vi "BT-Android_AE_sub.vi"(3 "port":u32=57600, 4 "file path (dialog if empty)":path=path "E:/测试数据/新芯片", 5 "mode":T1, 6 "timeout (10sec)":u32=10000, 7 "End Write on Termination Character?":bool, 8 "error in (no error)":errorcluster, 9 "存盘":bool, 10 "send data":string, 11 "VISA resource name":refnum<visa-resource-name>="COM13") -> (0 "error IO":errorcluster, 2 "timeout?":bool=TRUE)   [LabVIEW 2016, in "BT-Android_interface.lvlib"]
uses:
  BT-Android_interface.lvlib
  mode.ctl
  <vilib>/Utility/file.llb/Write Delimited Spreadsheet (I64).vi
  <vilib>/Instr/_visa.llb/VISA Configure Serial Port (Instr).vi
panel:
  in  "Termination Character":u8=10 format="%.0x"
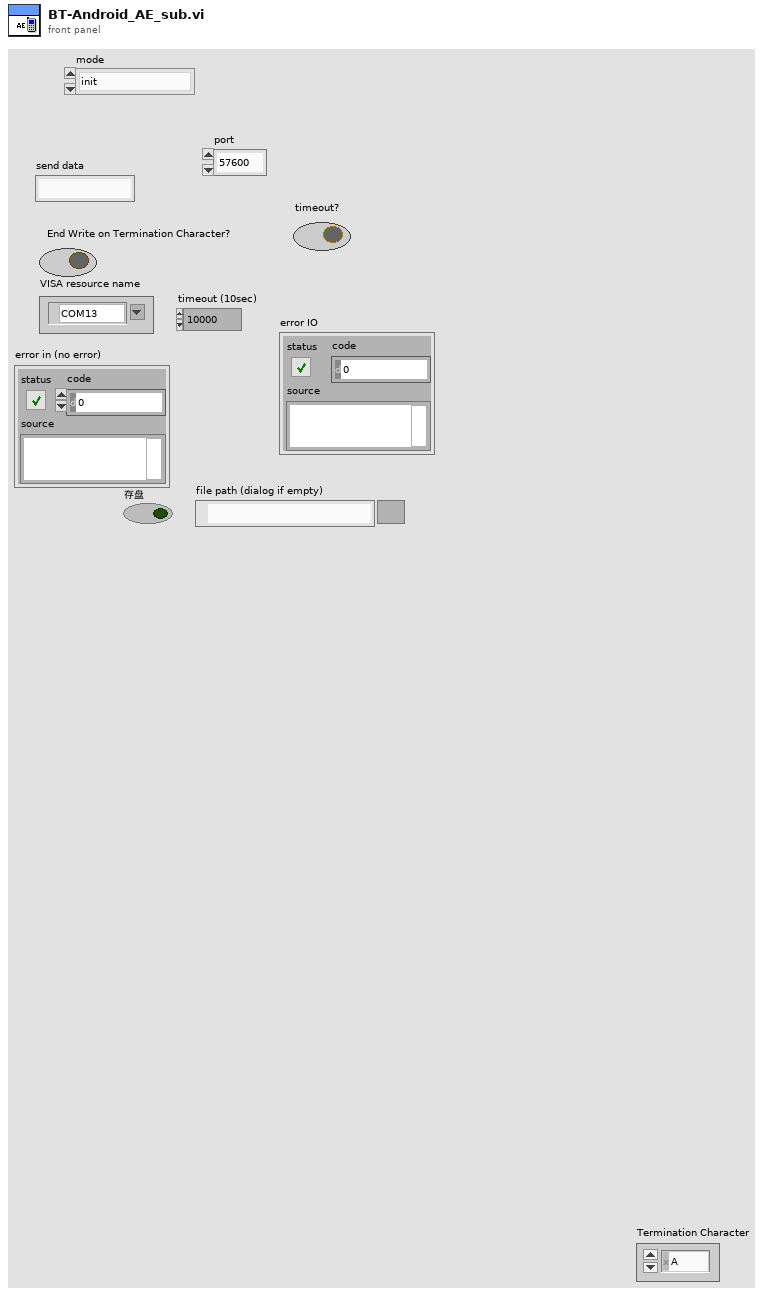
[diagram p1: front panel]
types:
  T1 = typedef "BT-Android_interface.lvlib/mode.ctl" = enum16{"init", "broadcast_data", "receive_data", "close"}
  T2 = enum16{"Standard", "Buffered", "CRLF", "Immediate"}
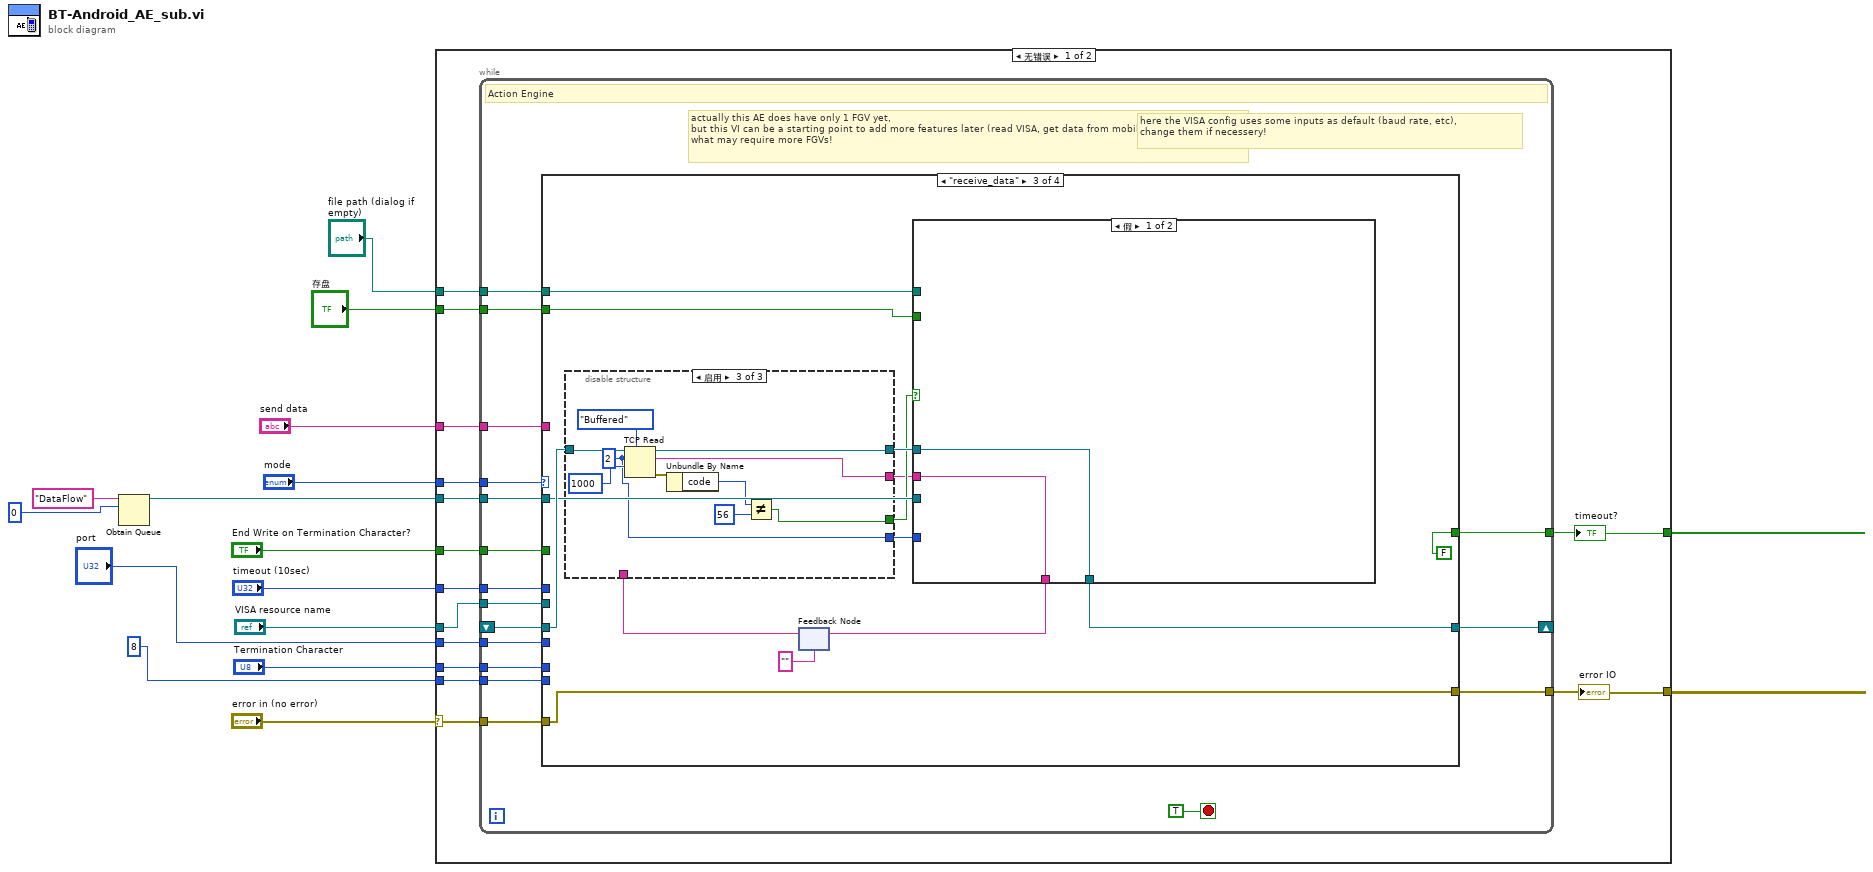
[diagram p0: block diagram]
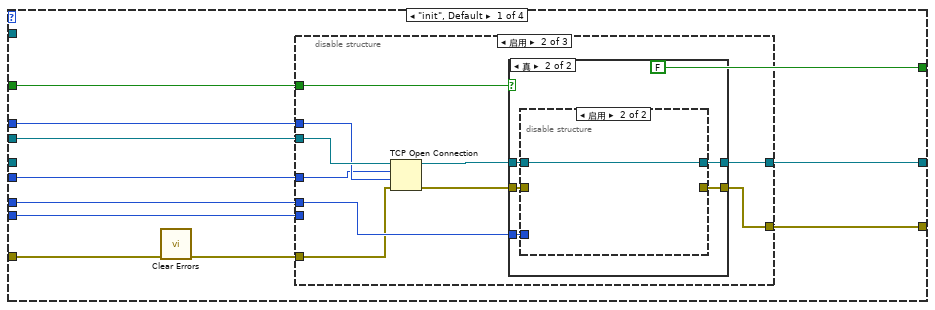
[diagram p2: hidden frame]
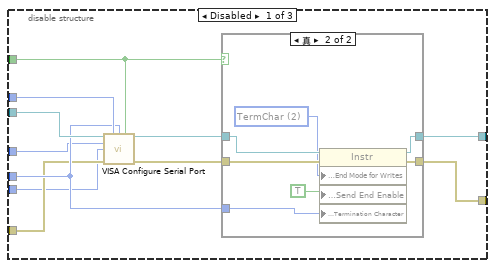
[diagram p3: hidden frame]
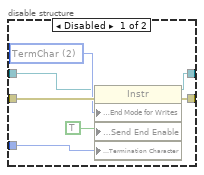
[diagram p6: hidden frame]
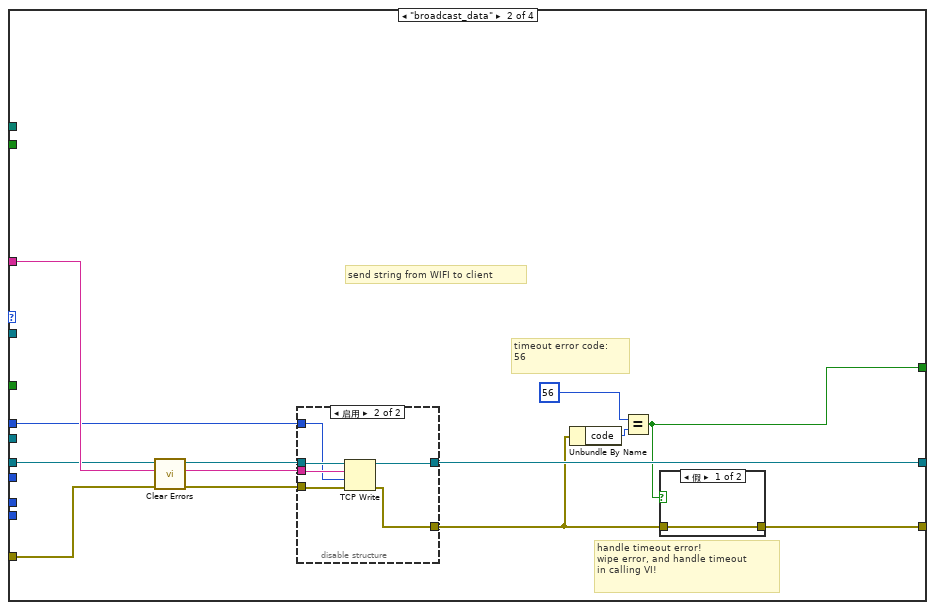
[diagram p8: hidden frame]
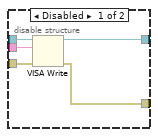
[diagram p9: hidden frame]
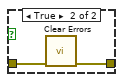
[diagram p10: hidden frame]
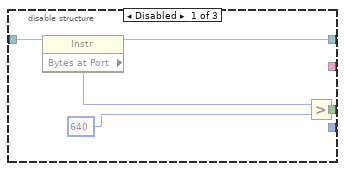
[diagram p11: hidden frame]
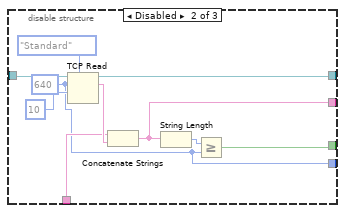
[diagram p12: hidden frame]
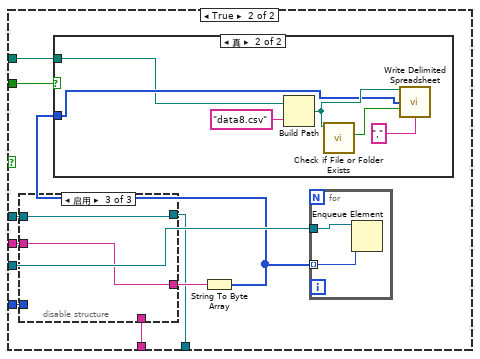
[diagram p13: hidden frame]
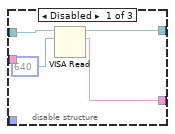
[diagram p14: hidden frame]
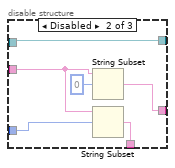
[diagram p15: hidden frame]
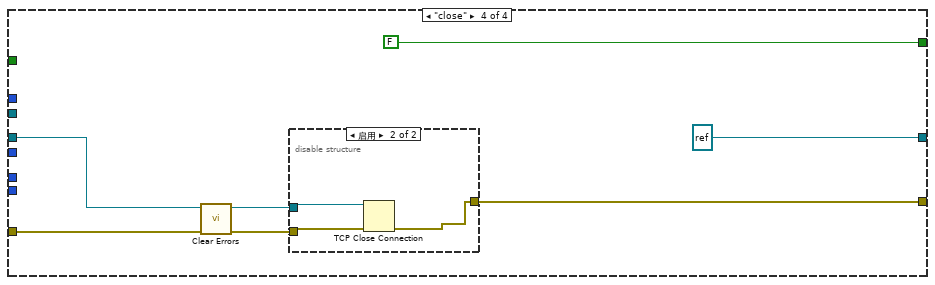
[diagram p17: hidden frame]
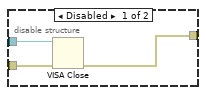
[diagram p18: hidden frame]
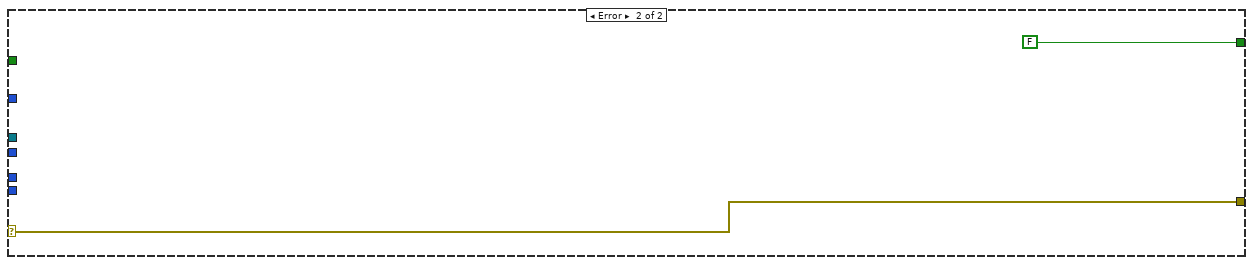
[diagram p19: hidden frame]
diagram:
  n1 = Obtain Queue(name (unnamed)="DataFlow", element data type=u8 0) -> (queue out=w5:refnum<queue>)  [unwired: 3 in, 2 out]
  n2 = case shown="无错误" "error in (no error)" {
    selector: "error in (no error)" -> [w30 w213]
    tunnel: [w26 w213] -> w15
    tunnel: "mode" -> [w29 _]
    tunnel: "End Write on Termination Character?" -> [w28 _]
    tunnel: "timeout (10sec)" -> [w27 _]
    tunnel: "VISA resource name" -> [w22 _]
    tunnel: "Termination Character" -> [w25 _]
    tunnel: "send data" -> [w24 _]
    tunnel: [w23 FALSE] -> w8
    tunnel: w5 -> [w21 _]
    tunnel: "port" -> [w20 _]
    tunnel: 8 -> [w19 _]
    tunnel: "存盘" -> [w18 _]
    tunnel: "file path (dialog if empty)" -> [w17 _]
    frame No Error {
      n3 = while {
        tunnel: w30 -> [w46]
        tunnel: w29 -> [w45]
        tunnel: w28 -> [w44]
        tunnel: w27 -> [w43]
        shift-right: [w42] -> _
        shift-left: _ -> [w36]
        tunnel: [w41] -> w26
        tunnel: w25 -> [w40]
        tunnel: w24 -> [w39]
        tunnel: [w38] -> w23
        tunnel: w22 -> [w37]
        tunnel: w21 -> [w35]
        tunnel: w20 -> [w34]
        tunnel: w19 -> [w33]
        tunnel: w18 -> [w32]
        tunnel: w17 -> [w31]
        stop <- TRUE stop-if-true
        # "here the VISA config uses some inputs as default (baud rate, etc),\nchange them if necessery!"
        # "actually this AE does have only 1 FGV yet, \nbut this VI can be a starting point to add more features later (read VISA, get data from mobile)\nwhat may require more FGVs!"
        # "Action Engine"
        n4 = case shown="\"receive_data\"" w45 {
          tunnel: w46 -> [w53 w114 w137 w205]
          tunnel: w44 -> [w51 _ _ _]
          tunnel: w43 -> [w58 w105 _ _]
          tunnel: w37 -> [w57 _ _ _]
          tunnel: [w56 w113 w138 refnum<k5> refnum ("connection ID")] -> w42
          tunnel: [w55 w111 w137 w204] -> w41
          tunnel: w40 -> [w54 _ _ _]
          tunnel: w39 -> [_ w112 _ _]
          tunnel: [FALSE w107 FALSE FALSE] -> w38
          tunnel: w36 -> [_ w106 w142 w201]
          tunnel: w35 -> [_ _ w140 _]
          tunnel: w34 -> [w50 _ _ _]
          tunnel: w33 -> [w49 _ _ _]
          tunnel: w32 -> [_ _ w136 _]
          tunnel: w31 -> [_ _ w135 _]
          frame "init", Default {
            n5 = call <vilib>:"Clear Errors.vi"("error in (no error)"=w53) -> ("error out"=w48:errorcluster)  [unwired: 5 in, 1 out]
            n6 = disable-structure shown="启用" {
              disable-tunnel: w58 -> [w67 w80 _]
              disable-tunnel: w57 -> [w66 w86 _]
              disable-tunnel: [w65 w85 _] -> w56
              disable-tunnel: [w64 w84 _] -> w55
              disable-tunnel: w54 -> [w63 w83 _]
              disable-tunnel: w48 -> [w62 w81 _]
              disable-tunnel: w51 -> [w61 w82 _]
              disable-tunnel: w50 -> [w60 w79 _]
              disable-tunnel: w49 -> [w59 _ _]
              frame Disabled {
                n7 = call-poly "VISA Configure Serial Port"("VISA resource name"=w66, "timeout (10sec)"=w67, "termination char\n(0xA = '\\n' = LF)"=w63, "Enable Termination\nChar (T)"=w61, "baud rate (9600)"=w60, "data bits (8)"=w59, "error in (no error)"=w62) -> ("VISA resource name out"=w68:refnum<visa-resource-name>, "error out"=w69:errorcluster)  [unwired: 3 in, 4 out]
                n8 = case shown="真" w61 {
                  tunnel: w68 -> [w70 w78]
                  tunnel: w69 -> [w71 w77]
                  tunnel: [w70 w76] -> w65
                  tunnel: [w71 w75] -> w64
                  tunnel: w63 -> [_ w73]
                  frame False {
                  }
                  frame True {
                    w74 = u16 2 items=["None", "LastBit", "TermChar", "Break"] ("Serial Settings:Serial End Mode for Writes")
                    n9 = property class="Instr"(reference=w78, error in=w77, "Serial Settings:End Mode for Writes"=w74, "Message Based Settings:Send End Enable"=TRUE, "Message Based Settings:Termination Character"=w73) -> (reference out=w76:refnum<visa-resource-name>, error out=w75:errorcluster)
                  }
                }
              }
              frame Enabled {
                n10 = TCP Open Connection(address=w86, remote port or service name=w79, timeout ms (60000)=w80, error in (no error)=w81) -> (connection ID=w87:refnum<k5>, error out=w88:errorcluster)  [unwired: 1 in]
                n11 = case shown="真" w82 {
                  tunnel: w87 -> [w89 w91]
                  tunnel: w88 -> [w90 w95]
                  tunnel: [w89 w94] -> w85
                  tunnel: [w90 w93] -> w84
                  tunnel: w83 -> [_ w92]
                  frame False {
                  }
                  frame True {
                    n12 = disable-structure shown="启用" {
                      disable-tunnel: w95 -> [w102 _]
                      disable-tunnel: [w101 w103] -> w94
                      disable-tunnel: [w100 _] -> w93
                      disable-tunnel: w92 -> [w98 _]
                      disable-tunnel: w91 -> [w96 w103]
                      frame Disabled {
                        w99 = u16 2 items=["None", "LastBit", "TermChar", "Break"] ("Serial Settings:Serial End Mode for Writes")
                        n13 = property class="Instr"(reference=w96, error in=w102, "Serial Settings:End Mode for Writes"=w99, "Message Based Settings:Send End Enable"=TRUE, "Message Based Settings:Termination Character"=w98) -> (reference out=w101:refnum<visa-resource-name>, error out=w100:errorcluster)
                      }
                      frame Enabled {
                      }
                    }
                  }
                }
              }
              frame Disabled {
              }
            }
          }
          frame "broadcast_data" {
            # "send string from WIFI to client"
            # "handle timeout error!\nwipe error, and handle timeout\nin calling VI!"
            # "timeout error code:\n56"
            n14 = call <vilib>:"Clear Errors.vi"("error in (no error)"=w114) -> ("error out"=w104:errorcluster)  [unwired: 5 in, 1 out]
            n15 = disable-structure shown="启用" {
              disable-tunnel: w104 -> [w119 w124]
              disable-tunnel: [w118 w122] -> w113
              disable-tunnel: w112 -> [w117 w123]
              disable-tunnel: [w116 w121] -> w110
              disable-tunnel: w106 -> [w115 w125]
              disable-tunnel: w105 -> [_ w120]
              frame Disabled {
                n16 = VISA Write(VISA resource name=w115, write buffer=w117, error in (no error)=w119) -> (VISA resource name out=w118:refnum<visa-resource-name>, error out=w116:errorcluster)  [unwired: 1 out]
              }
              frame Enabled {
                n17 = TCP Write(connection ID=w125, data in=w123, error in (no error)=w124, 9:w120) -> (connection ID out=w122:refnum<k5>, error out=w121:errorcluster)  [unwired: 1 out]
              }
            }
            n18 = Unbundle By Name(w110) -> ("code"=w109:i32)
            n19 = Equal?(x=56 ("code"), y=w109) -> (x = y?=w107:bool)
            n20 = case shown="假" w107 {
              tunnel: w110 -> [w126 w128]
              tunnel: [w126 w127] -> w111
              frame False {
              }
              frame True {
                n21 = call <vilib>:"Clear Errors.vi"("error in (no error)"=w128) -> ("error out"=w127:errorcluster)  [unwired: 5 in, 1 out]
              }
            }
          }
          frame "receive_data" {
            n22 = feedback #1("") -> (w132:string)
            n23 = disable-structure shown="启用" {
              disable-tunnel: w142 -> [w147 w157 w167]
              disable-tunnel: [w146 w155 w165] -> w141
              disable-tunnel: [w143 w150 w159] -> w134
              disable-tunnel: w132 -> [_ w151 _]
              disable-tunnel: [_ w149 w162] -> w131
              disable-tunnel: [_ w148 w163] -> w130
              frame Disabled {
                n24 = property class="Instr"(reference=w147) -> (reference out=w146:refnum<visa-resource-name>, "Bytes at Port"=w145:u32)  [unwired: 1 in, 1 out]
                n25 = Greater?(x=w145, y=640) -> (0:w143:bool)
              }
              frame Disabled {
                w148 = 640 ("读取的字节")
                n26 = TCP Read(connection ID=w157, bytes to read=w148, 7:T2."Standard" ("模式（标准）"), 9:10 ("超时毫秒(25000)")) -> (connection ID out=w155:refnum<k5>, data out=w152:string)  [unwired: 1 in, 1 out]
                n27 = Concatenate Strings(w151, w152) -> (w149:string)
                n28 = String Length(string=w149) -> (length=w153:i32)
                n29 = Greater Or Equal?(x=w153, y=w148) -> (x >= y?=w150:bool)
              }
              frame Enabled {
                w163 = 2 ("读取的字节")
                n30 = TCP Read(connection ID=w167, bytes to read=w163, 7:T2."Buffered" ("模式（标准）"), 9:1000 ("超时毫秒(25000)")) -> (connection ID out=w165:refnum<k5>, data out=w162:string, error out=w161:errorcluster)  [unwired: 1 in]
                n31 = Unbundle By Name(w161) -> ("code"=w160:i32)
                n32 = Not Equal?(x=w160, y=56) -> (x != y?=w159:bool)
              }
            }
            n33 = case shown="假" w134 {
              tunnel: w141 -> [w169 w179]
              tunnel: w140 -> [_ w177]
              tunnel: [w169 w176] -> w138
              tunnel: w136 -> [_ w175]
              tunnel: w135 -> [_ w174]
              tunnel: w131 -> [w168 w172]
              tunnel: w130 -> [_ w171]
              tunnel: [w168 w170] -> w129
              frame False {
              }
              frame True {
                n34 = disable-structure shown="启用" {
                  disable-tunnel: w179 -> [w183 w189 w191]
                  disable-tunnel: [w182 w185 w190] -> w178
                  disable-tunnel: [w181 w189 w191] -> w176
                  disable-tunnel: w172 -> [_ w187 w190]
                  disable-tunnel: w171 -> [_ w186 _]
                  disable-tunnel: [_ w184 _] -> w170
                  frame Disabled {
                    n35 = VISA Read(VISA resource name=w183, byte count=640) -> (VISA resource name out=w181:refnum<visa-resource-name>, read buffer=w182:string)  [unwired: 1 in, 2 out]
                  }
                  frame Disabled {
                    n36 = String Subset(string=w187, offset (0)=0 ("偏移量(0)")) -> (substring=w185:string)  [unwired: 1 in]
                    n37 = String Subset(string=w187, offset (0)=w186) -> (substring=w184:string)  [unwired: 1 in]
                  }
                  frame Enabled {
                  }
                }
                n38 = String To Byte Array(string=w178) -> (unsigned byte array=w173:u8[])
                n39 = case shown="真" w175 {
                  tunnel: w173 -> [_ w193]
                  tunnel: w174 -> [_ w192]
                  frame False {
                  }
                  frame True {
                    n40 = Build Path(base path=w192, name or relative path="data8.csv") -> (appended path=w194:path)
                    n41 = call <vilib>:"Check if File or Folder Exists.vi"("path"=w194) -> ("file or folder exists?"=w197:bool)  [unwired: 8 in, 2 out]
                    n42 = call-poly <vilib>:"Write Delimited Spreadsheet.vi"("file path (dialog if empty)"=w194, "1D data"=w193, "append to file? (new file:F)"=w197, "delimiter (\\t)"="," ("delimiter (\\t)")) -> ()  [unwired: 10 in, 2 out]
                  }
                }
                n43 = for {
                  tunnel: w173 -> [w199] mode=indexing
                  tunnel: w177 -> [w198]
                  n44 = Enqueue Element(queue=w198, element=w199) -> ()  [unwired: 2 in, 3 out]
                }
              }
            }
            n45 = feedback-in #1(w129) -> ()
          }
          frame "close" {
            n46 = call <vilib>:"Clear Errors.vi"("error in (no error)"=w205) -> ("error out"=w200:errorcluster)  [unwired: 5 in, 1 out]
            n47 = disable-structure shown="启用" {
              disable-tunnel: w200 -> [w208 w210]
              disable-tunnel: [w207 w209] -> w204
              disable-tunnel: w201 -> [w206 w211]
              frame Disabled {
                n48 = VISA Close(VISA resource name=w206, error in (no error)=w208) -> (error out=w207:errorcluster)
              }
              frame Enabled {
                n49 = TCP Close Connection(connection ID=w211, error in (no error)=w210) -> (error out=w209:errorcluster)  [unwired: 1 in, 1 out]
              }
            }
          }
        }
      }
    }
    frame Error {
    }
  }
  "error IO" <- w15
  "timeout?" <- w8
